vi "ShooterNoPID.vi"(5 "WinchCaseIn":i32, 8 "InGearPosLow":dbl=1.5, 9 "InGearPosHigh":dbl=2.1, 10 "Pot":dbl, 11 "Fire":bool) -> (0 "There?":bool, 1 "WinchCase":i32, 3 "Power":dbl)   [LabVIEW 2013]
panel:
  out "Index":i32
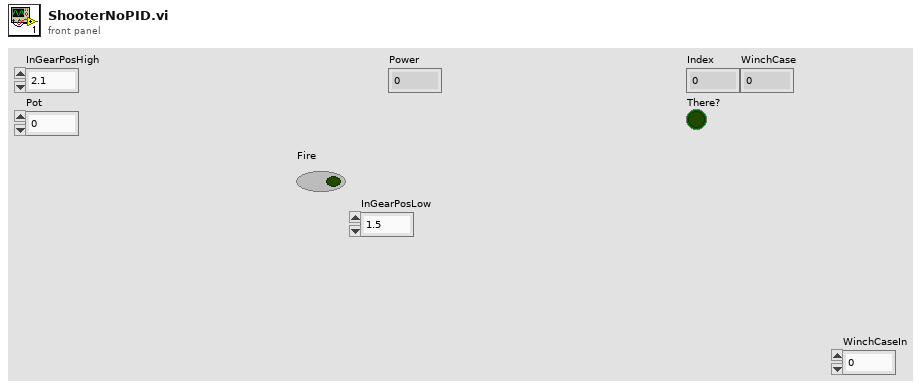
[diagram p1: front panel]
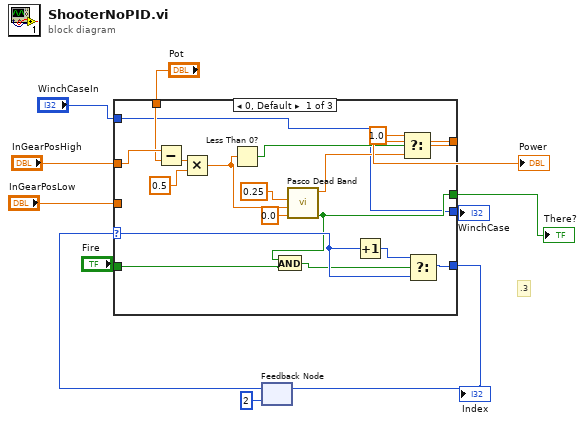
[diagram p0: block diagram]
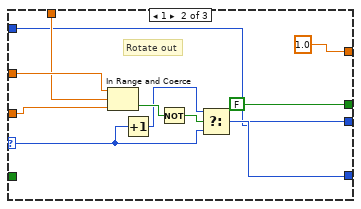
[diagram p2: hidden frame]
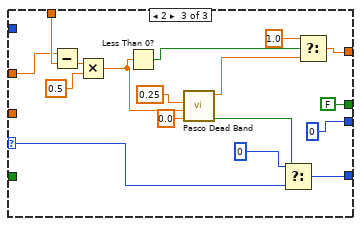
[diagram p3: hidden frame]
diagram:
  # ".3"
  n1 = feedback #1(2 ("Numeric")) -> (w9:i32)
  n2 = case shown="0, Default" w9 {
    selector: w9 -> [w29 w34 w44]
    tunnel: [w12 1.0 ("Output") w52] -> w3
    tunnel: "Fire" -> [w16 _ _]
    tunnel: [w27 w33 w43] -> w1
    tunnel: "InGearPosHigh" -> [w18 w40 w56]
    tunnel: "InGearPosLow" -> [_ w39 _]
    tunnel: "Pot" -> [w17 w38 w57]
    tunnel: [w13 w32 0] -> w5
    tunnel: "WinchCaseIn" -> [w13 w32 _]
    tunnel: [w14 FALSE FALSE] -> w2
    frame 0, Default {
      n3 = Subtract(x=w18, y=w17) -> (x-y=w26:dbl)
      n4 = Multiply(x=w26, y=0.5) -> (x*y=w22:dbl)
      n5 = Less Than 0?(x=w22) -> (x < 0?=w24:bool)
      n6 = call "Pasco Dead Band.vi"("lower limit"=0.0, "PWM Power"=w22, "upper limit"=0.25) -> ("Integral Reset"=w14:bool, "PWM Power"=w19:dbl)  [unwired: 7 in]
      n7 = And(x=w14, y=w16) -> (x .and. y?=w15:bool)
      n8 = Increment(x=w29) -> (x+1=w28:i32)
      n9 = Select(t=1.0, s=w24, f=w19) -> (s? t:f=w12:dbl)
      n10 = Select(t=w28, s=w15, f=w29) -> (s? t:f=w27:i32)
    }
    frame 1 {
      # "Rotate out"
      n11 = In Range and Coerce(upper limit=w40, x=w38, lower limit=w39) -> (In Range?=w37:bool)  [unwired: 1 out]
      n12 = Increment(x=w34) -> (x+1=w35:i32)
      n13 = Not(x=w37) -> (.not. x?=w36:bool)
      n14 = Select(t=w35, s=w36, f=w34) -> (s? t:f=w33:i32)
    }
    frame 2 {
      n15 = Subtract(x=w56, y=w57) -> (x-y=w55:dbl)
      n16 = Multiply(x=w55, y=0.5) -> (x*y=w50:dbl)
      n17 = Less Than 0?(x=w50) -> (x < 0?=w53:bool)
      n18 = call "Pasco Dead Band.vi"("lower limit"=0.0, "PWM Power"=w50, "upper limit"=0.25) -> ("Integral Reset"=w46:bool, "PWM Power"=w47:dbl)  [unwired: 7 in]
      n19 = Select(t=0, s=w46, f=w44) -> (s? t:f=w43:i32)
      n20 = Select(t=1.0, s=w53, f=w47) -> (s? t:f=w52:dbl)
    }
  }
  "Power" <- w3
  "Index" <- w1
  "There?" <- w2
  "WinchCase" <- w5
  n21 = feedback-in #1(w1) -> ()
